vi "Editor Tester.vi"() -> ()   [LabVIEW 2015]
uses:
  Forms/Rectangle/Rectangle.lvclass
  Forms/Line/Line.lvclass
  Image Editor Handler/Image Editor Handler.lvclass
  Forms/Shape/Shape.lvclass/Shape.ctl
  Forms/Rectangle/Rectangle.lvclass/Rectangle.ctl
  Forms/Layered Shape/Layered Shape.lvclass/Layered Shape.ctl
  Forms/Shape/Write Color.vi
  Forms/Rectangle/Write Filled.vi
  Forms/Layered Shape/Write Overlays.vi
  Forms/Text/Text.lvclass
  Forms/Shape/Shape.lvclass
  Forms/Link/Link.lvclass
panel:
  in  "2D Picture":picture
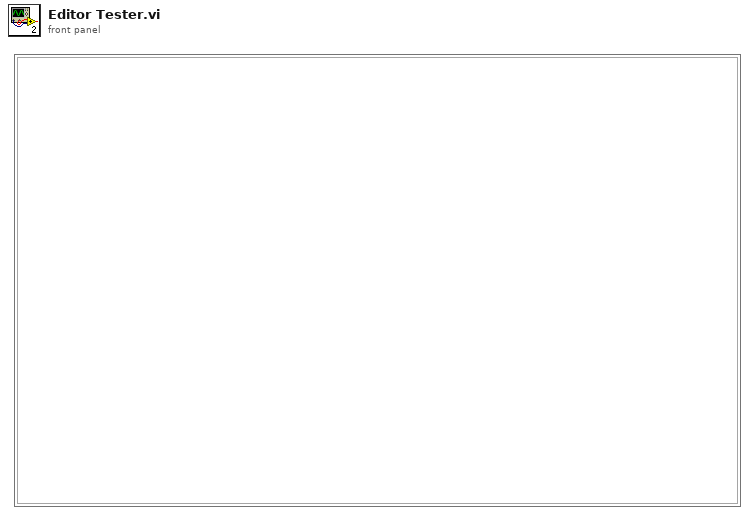
[diagram p1: front panel]
types:
  T1 = cluster{"Font Name:":string, "Size":i16, "Strikeout?":bool, "Italic?":bool, "Underline?":bool, "Outline?":bool, "Shadow?":bool, "Bold?":bool}
  T2 = cluster{"Width":u16, "Style":enum32{"Solid", "Dash", "Dot", "DashDot", "DashDotDot"}}
  T3 = enum16{"Left", "Top", "Right", "Bottom", "Centered"}
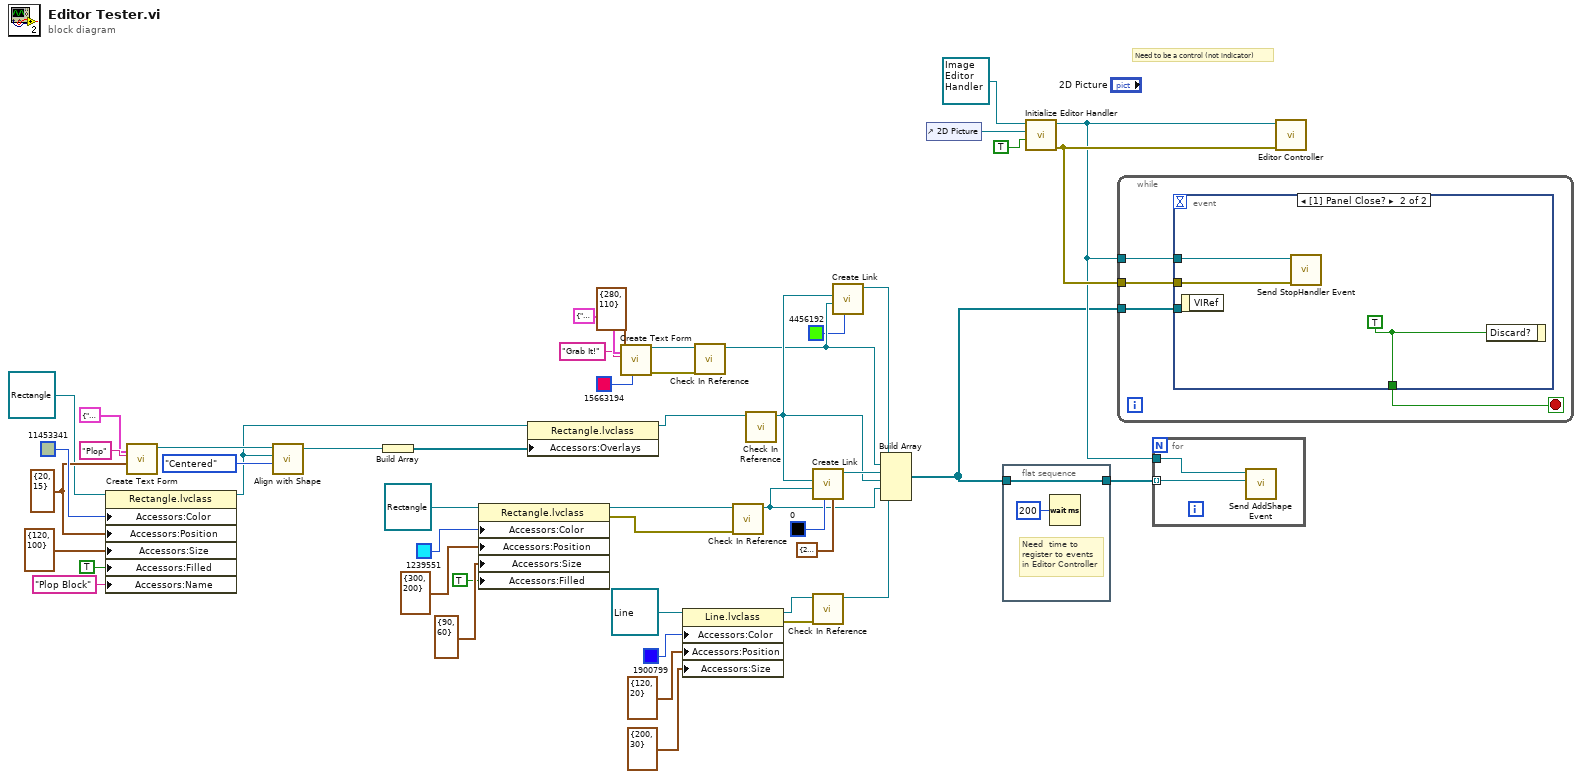
[diagram p0: block diagram]
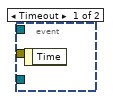
[diagram p2: hidden frame]
diagram:
  w33 = cluster{"Left":i32, "Top":i32} {"Left"=20, "Top"=15} ("Position")
  # "Need to be a control (not indicator)"
  n1 = property class="Rectangle.lvclass"(reference=refnum<class "Rectangle.lvclass"> refnum ("Rectangle.lvclass"), "Accessors:Color"=u32 11453341 ("Color"), "Accessors:Position"=w33, "Accessors:Size"=cluster{"Width":i32, "Height":i32} {"Width"=120, "Height"=100} ("Size"), "Accessors:Filled"=TRUE ("Filled"), "Accessors:Name"="Plop Block" ("Name")) -> (reference out=w25:refnum<class "Rectangle.lvclass">)  [unwired: 1 in, 1 out]
  n2 = call "Create Text Form.vi"("[user-specified font]"=T1 {"Font Name:"="SegoeUI", "Size"=18, "Strikeout?"=FALSE, "Italic?"=FALSE, "Underline?"=FALSE, "Outline?"=FALSE, "Shadow?"=FALSE, "Bold?"=TRUE}, "Origin"=w33, "Text"="Plop") -> ("New Text"=w26:refnum<class "Text.lvclass">)  [unwired: 7 in, 1 out]
  n3 = call "Align with Shape.vi"("Alignment"=T3."Centered", "Reference Shape"=w25, "Shape in"=w26) -> ("Shape out"=w2:refnum<class "Text.lvclass">)  [unwired: 7 in, 1 out]
  n4 = Build Array(w2) -> (w1:refnum<class "Text.lvclass">[])
  n5 = property class="Rectangle.lvclass"(reference=refnum<class "Rectangle.lvclass"> refnum ("Rectangle.lvclass"), "Accessors:Color"=u32 1239551 ("Color"), "Accessors:Position"=cluster{"Left":i32, "Top":i32} {"Left"=300, "Top"=200} ("Position"), "Accessors:Size"=cluster{"Width":i32, "Height":i32} {"Width"=90, "Height"=60} ("Size"), "Accessors:Filled"=TRUE ("Filled")) -> (reference out=w40:refnum<class "Rectangle.lvclass">, error out=w41:errorcluster)  [unwired: 1 in]
  n6 = property class="Rectangle.lvclass"(reference=w25, "Accessors:Overlays"=w1) -> (reference out=w28:refnum<class "Rectangle.lvclass">)  [unwired: 1 in, 1 out]
  n7 = call "Create Text Form.vi"("Color"=u32 15663194, "[user-specified font]"=T1 {"Font Name:"="SegoeUI", "Size"=24, "Strikeout?"=FALSE, "Italic?"=FALSE, "Underline?"=TRUE, "Outline?"=FALSE, "Shadow?"=FALSE, "Bold?"=TRUE}, "Origin"=cluster{"horizontal":i16, "vertical":i16} {"horizontal"=280, "vertical"=110}, "Text"="Grab It!") -> ("error out"=w12:errorcluster, "New Text"=w13:refnum<class "Text.lvclass">)  [unwired: 6 in]
  n8 = property class="Line.lvclass"(reference=refnum<class "Line.lvclass"> refnum ("Line.lvclass"), "Accessors:Color"=u32 1900799 ("Color"), "Accessors:Position"=cluster{"Left":i32, "Top":i32} {"Left"=120, "Top"=20} ("Position"), "Accessors:Size"=cluster{"Width":i32, "Height":i32} {"Width"=200, "Height"=30} ("Size")) -> (reference out=w35:refnum<class "Line.lvclass">, error out=w29:errorcluster)  [unwired: 1 in]
  n9 = call "Check In Reference.vi"("error in (no error)"=w12, "Shape in"=w13) -> ("Shape Reference"=w7:refnum<data-value>)  [unwired: 8 in, 1 out]
  n10 = call "Check In Reference.vi"("error in (no error)"=w41, "Shape in"=w40) -> ("Shape Reference"=w18:refnum<data-value>)  [unwired: 8 in, 1 out]
  n11 = call "Check In Reference.vi"("Shape in"=w28) -> ("Shape Reference"=w8:refnum<data-value>)  [unwired: 9 in, 1 out]
  n12 = call "Create Link.vi"("Style"=T2 {"Width"=2, "Style"=enum."Solid"}, "Color"=u32 0, "Destination"=w18, "Source"=w8) -> ("Link Reference"=w19:refnum<data-value>)  [unwired: 6 in, 1 out]
  n13 = call "Check In Reference.vi"("error in (no error)"=w29, "Shape in"=w35) -> ("Shape Reference"=w17:refnum<data-value>)  [unwired: 8 in, 1 out]
  n14 = call "Create Link.vi"("Color"=u32 4456192, "Destination"=w7, "Source"=w8) -> ("Link Reference"=w6:refnum<data-value>)  [unwired: 7 in, 1 out]
  n15 = Build Array(w6, w7, w19, w8, w18, w17) -> (w10:refnum<data-value>[])
  n16 = control-ref of="2D Picture"() -> (w49:refnum<vi>)
  n17 = flat-sequence {
    tunnel: w10 -> [w50]
    tunnel: [w50] -> w9
    frame #0 {
      # "Need  time to register to events in Editor Controller"
      n18 = Wait (ms)(milliseconds to wait=u32 200) -> ()  [unwired: 1 out]
    }
  }
  n19 = call "Initialize Editor Handler.vi"("Clear Picture?"=TRUE ("Clean Picture?"), "PictureRef"=w49, "Editor Handler in"=refnum<class "Image Editor Handler.lvclass"> refnum) -> ("error out"=w48:errorcluster, "Editor Handler out"=w47:refnum<class "Image Editor Handler.lvclass">)  [unwired: 6 in, 1 out]
  n20 = while {
    tunnel: w48 -> [w53]
    tunnel: w47 -> [w55]
    tunnel: w10 -> [w52]
    stop <- w54 stop-if-true
    n21 = event shown="[1] Panel Close?" {
      selector: _ -> [_ _]
      dyn-events: _ -> [_ _]
      timeout: _ -> [_ _]
      tunnel: w55 -> [_ w57]
      tunnel: [_ w58] -> w54
      tunnel: w53 -> [_ w56]
      tunnel: w52 -> [_ _]
      event Timeout {
        n22 = event-data() -> ()  [unwired: 1 in, 1 out]
      }
      event Panel Close? {
        w58 = TRUE ("Discard?")
        n23 = event-data() -> ()  [unwired: 1 in, 1 out]
        n24 = call "Send StopHandler Event.vi"("error in (no error)"=w56, "Editor Handler in"=w57) -> ()  [unwired: 8 in, 2 out]
        n25 = event-data("Discard?"=w58) -> ()  [unwired: 1 in, 1 out]
      }
    }
  }
  n26 = for {
    tunnel: w9 -> [w59] mode=indexing
    tunnel: w47 -> [w60]
    n27 = call "Send AddShape Event.vi"("New Shape Reference"=w59, "Editor Handler in"=w60) -> ()  [unwired: 8 in, 2 out]
  }
  n28 = call "Editor Controller.vi"("error in (no error)"=w48, "Editor Handler in"=w47) -> ()  [unwired: 8 in, 2 out]
